vi "Main.vi"() -> ()   [LabVIEW 2015]
doc: "本模板用于队列消息处理器设计模式。\n\n事件处理循环负责按用户界面操作生成对应的消息。\n\n消息处理循环负责对事件处理循环或其他消息生成的消息进行处理。消息内容为字符串值，因此很容易将新消息添加至“消息处理”循环的“消息分支”条件结构。每个消息簇还可选择性地为消息数据提供一个变体，变体数据可以转换为消息数据所需要的任意类型。"
uses:
  controls/UI Data.ctl
  <vilib>/Platform/TimedLoop/XDataNode/timing_clust.ctl
  <vilib>/Platform/TimedLoop/XDataNode/nitl_modes.ctl
  <vilib>/Platform/TimedLoop/XDataNode/wakeup.ctl
  support/Message Queue/Enqueue Message (Single).vi
  <vilib>/Utility/file.llb/Read Delimited Spreadsheet (string).vi
  <vilib>/Utility/error.llb/Error Cluster From Error Code.vi
  <vilib>/Platform/TimedLoop/XDataNode/XDataNode.xnode
  <vilib>/ErrorRing/Error Ring.xnode
  support/Message Queue/Message Queue.lvlib
  support/User Event - Stop/User Event - Stop.lvlib
  <vilib>/Platform/TimedLoop/XDataNode/XDNodeRunTimeDep.lvlib
panel:
  in  "选项卡控件":enum32{"总线检查", "报告生成"}(tab)
  in  "总线检查":bool
  in  "1560":refnum<visa-resource-name>="COM3"
  in  "目标温度":string(combo)
  in  "样品编号":string
  in  "生成报告":bool
  in  "误差计算":bool
  in  "均匀性测量":bool
  in  "位置":enum16{"A", "B", "C", "D", "E", "F", "G", "H"}(ring)
  in  "均匀性表格":string[][](table)=[["A", "O", "E", "O"], ["", "", "", ""], ["", "", "", ""], ["", "", "", ""], ["", "", "", ""], ["", "", "", ""], ["", "", "", ""], ["B", "O", "F", "O"], ["", "", "", ""], ["", "", "", ""], ["", "", "", ""], ["", "", "", ""], ["", "", "", ""], ["", "", "", ""], ["C", "O", "G", "O"], ["", "", "", ""], ["", "", "", ""], ["", "", "", ""], ["", "", "", ""], ["", "", "", ""], ["", "", "", ""], ["D", "O", "H", "O"], ["", "", "", ""], ["", "", "", ""], ["", "", "", ""], ["", "", "", ""], ["", "", "", ""], ["", "", "", ""], ["", "", "", ""], ["", "", "", ""]]
  in  "波动性表格":string[][](table)
  out "显示<替换该项>":string
  in  "波动性测量":bool
  in  "退出":bool
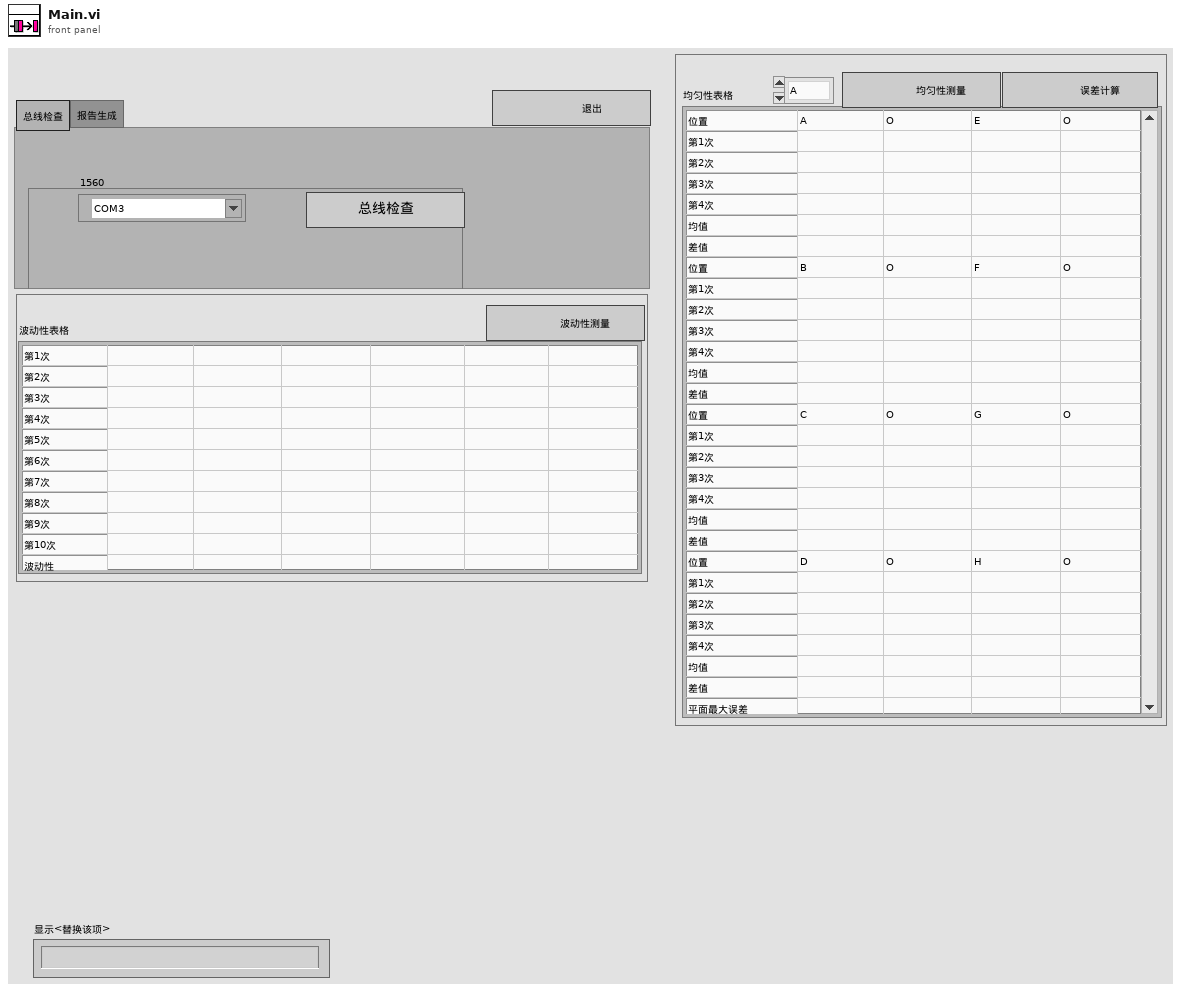
[diagram p1: front panel]
types:
  T1 = typedef "UI Data.ctl" = cluster{"布尔<替换该项>":bool, "字符串<替换该项>":string, "数值<替换该项>":dbl, "执行某操作引用":refnum<vi>, "执行其他操作引用":refnum<vi>, "数据显示引用":refnum<vi>, "退出按钮引用":refnum<vi>}
  T2 = typedef "Message Queue.lvlib/All Message Queues.ctl" = cluster{"UI":refnum<queue>}
  T3 = cluster{"Baud Rate (9600)":u32, "Flow Control (1: XON/XOFF)":u16, "Termination Char (0:CR)":u16}
  T4 = typedef "XDNodeRunTimeDep.lvlib/timing_clust.ctl" = cluster{"Expected End [f-1]":u64, "Actual End [f-1]":u64, "Finished Late? [f-1]":bool, "Expected End [i-1]":u64, "Actual End [i-1]":u64, "Finished Late? [i-1]":bool, "Expected Start [i]":u64, "Actual Start [i]":u64, "Expected Start [f]":u64, "Actual Start [f]":u64, "Source Name":string, "Structure Name":string, "Period":i64, "Deadline":i64, "Offset":i64, "Start":i64, "Priority":i32, "Timeout":i32, "Mode":T5, "Wakeup Reason":T6, "Error":errorcluster, "Source Type":string, "Secondary Source Type":string, "Global End Time":u64, "Global Start Time":u64, "Frame Duration":u64, "Iteration Duration":u64, "Assigned CPU":i32, "I/O Scan Engine Mode":u32}
  T5 = typedef "XDNodeRunTimeDep.lvlib/nitl_modes.ctl" = enum32{"No Change", "Process missed periods, maintain original phase", "Discard missed periods, maintain original phase", "Process missed periods, ignore original phase", "Discard missed periods, ignore original phase"}
  T6 = typedef "XDNodeRunTimeDep.lvlib/wakeup.ctl" = enum32{"Normal", "Aborted", "Asynchronous wakeup", "Timing source error", "Timed loop error", "Timeout"}
  T7 = enum8{"Enabled", "Disabled", "Disabled and Grayed Out"}
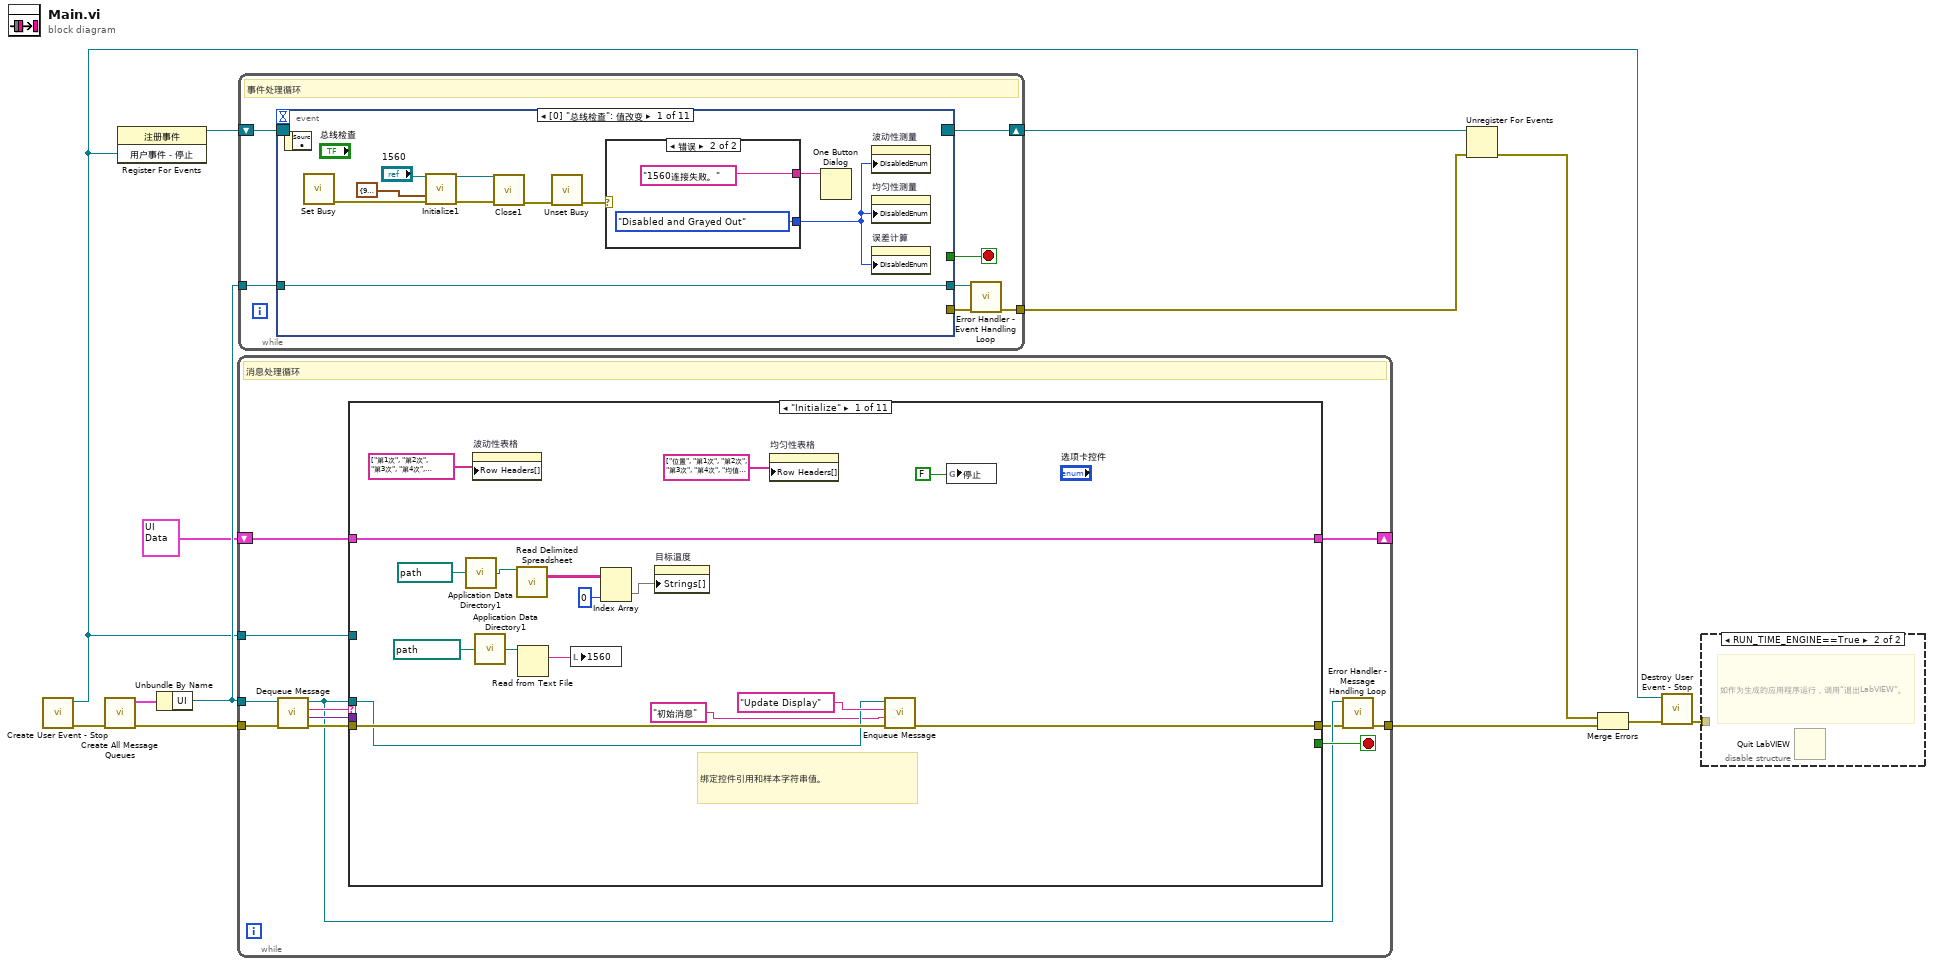
[diagram p0: block diagram]
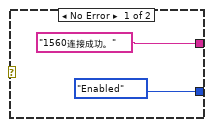
[diagram p3: hidden frame]
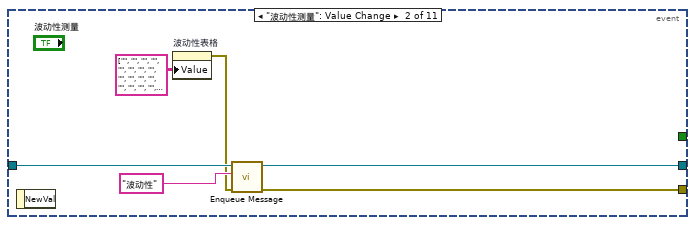
[diagram p4: hidden frame]
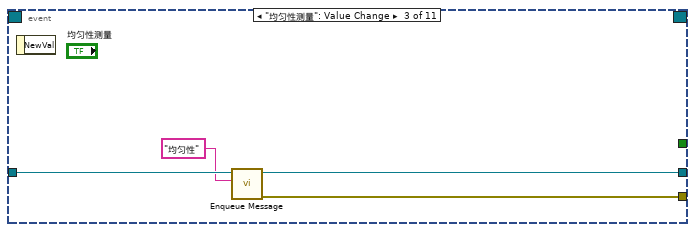
[diagram p5: hidden frame]
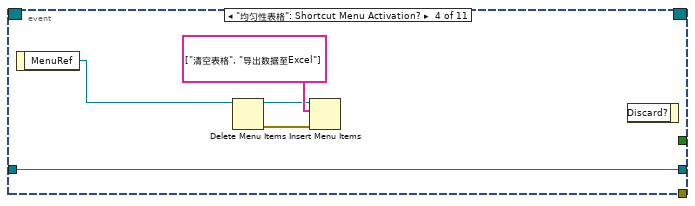
[diagram p6: hidden frame]
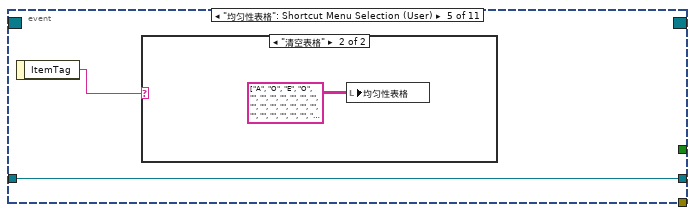
[diagram p7: hidden frame]
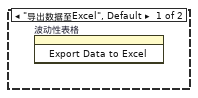
[diagram p8: hidden frame]
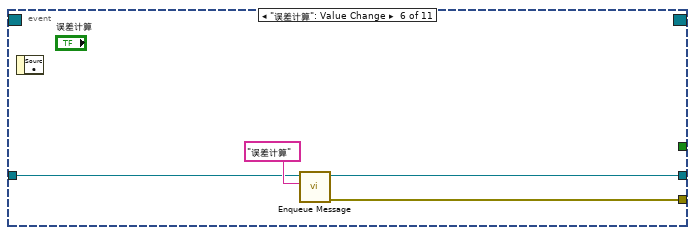
[diagram p9: hidden frame]
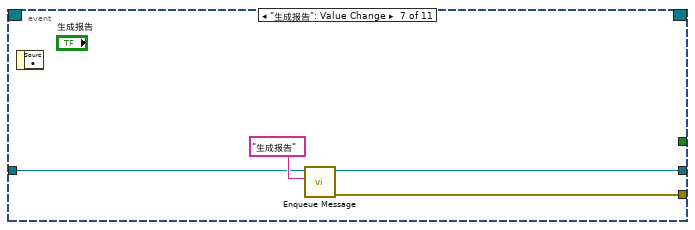
[diagram p10: hidden frame]
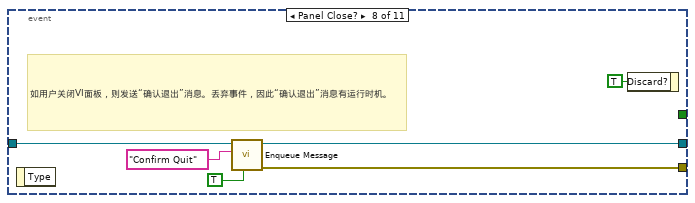
[diagram p11: hidden frame]
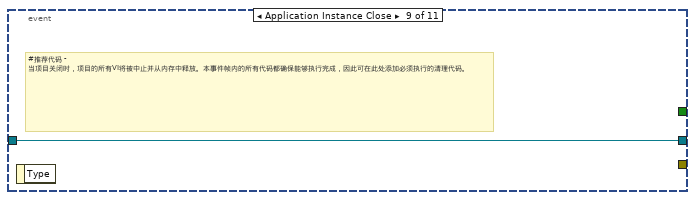
[diagram p12: hidden frame]
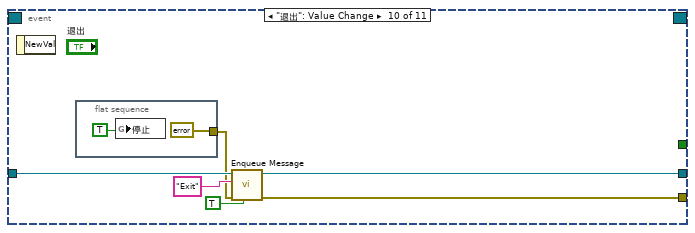
[diagram p13: hidden frame]
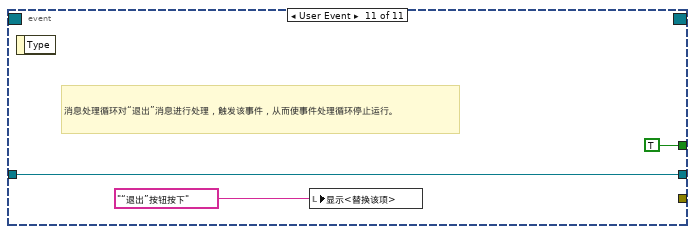
[diagram p14: hidden frame]
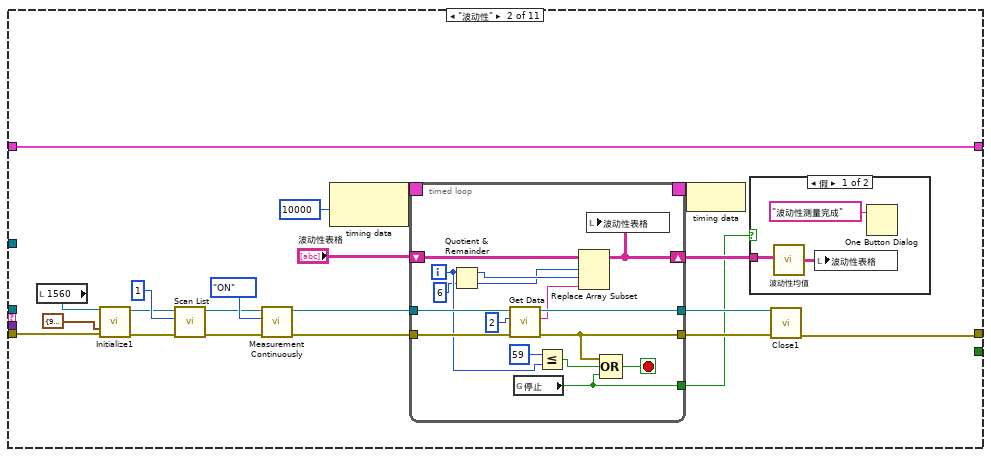
[diagram p15: hidden frame]
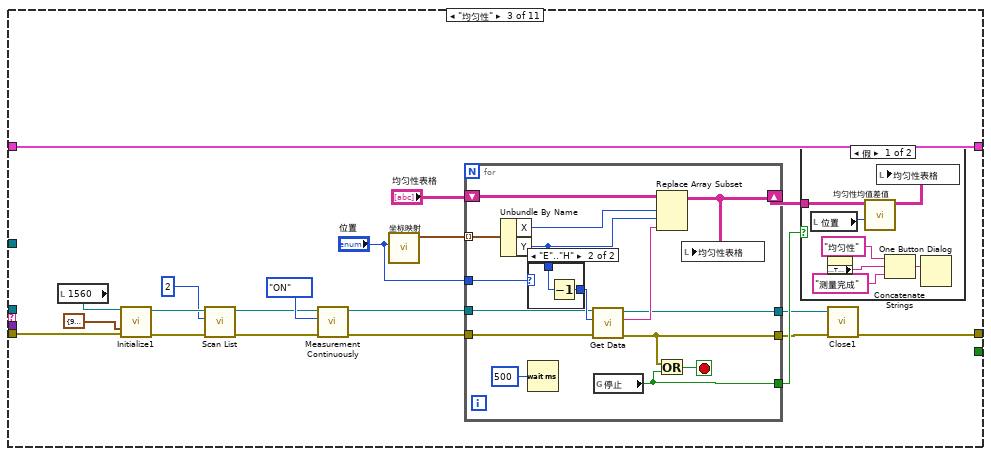
[diagram p17: hidden frame]
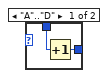
[diagram p19: hidden frame]
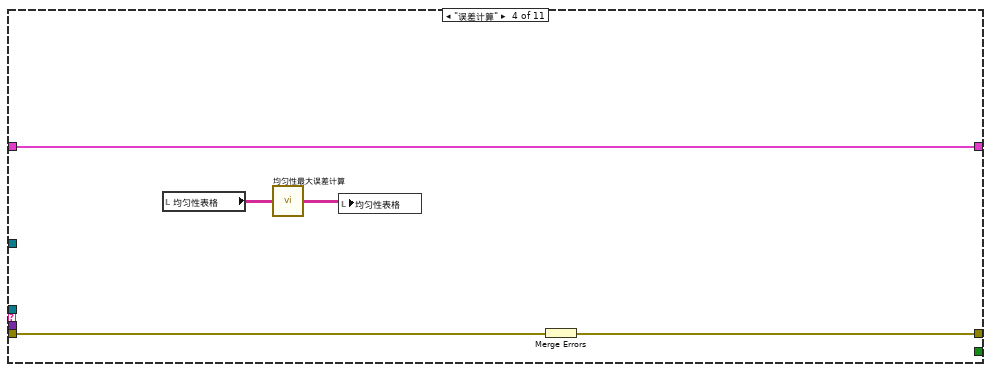
[diagram p20: hidden frame]
diagram:
  n1 = call "Create User Event - Stop.vi"() -> ("error out"=w9:cluster{"状态":bool, "代码":i32, "源":string}, "用户事件－停止"=w1:refnum<user-event>)  [unwired: 10 in]
  n2 = call "Create All Message Queues.vi"("error in (no error)"=w9) -> ("error out"=w13:cluster{"状态":bool, "代码":i32, "源":string}, "消息队列输出"=w12:T2)  [unwired: 9 in]
  n3 = register-events(w1) -> (reference out=w2:refnum<event-registration>)  [unwired: 2 in, 1 out]
  n4 = Unbundle By Name(w12) -> ("UI"=w10:refnum<queue>)
  n5 = while {
    tunnel: w10 -> [w17]
    shift-right: [w24] -> _
    shift-left: T1 {"布尔<替换该项>"=FALSE, "字符串<替换该项>"="", "数值<替换该项>"=0.0, "执行某操作引用"=refnum, "执行其他操作引用"=refnum, "数据显示引用"=refnum, "退出按钮引用"=refnum} ("Data Cluster") -> [w25]
    tunnel: w1 -> [w22]
    tunnel: w13 -> [w21]
    tunnel: [w15] -> w11
    stop <- w23 stop-if-true
    # "消息处理循环"
    n6 = call "Dequeue Message.vi"("error in (no error)"=w21, "消息队列"=w17) -> ("error out"=w20:cluster{"状态":bool, "代码":i32, "源":string}, "消息数据"=w18:variant, "消息"=w19:string, "消息队列副本"=w16:refnum<queue>)  [unwired: 6 in]
    n7 = case "消息分支" shown="\"Initialize\"" w19 {
      selector: w19 -> [_ _ _ _ _ _ _ _ _ _ w200]
      tunnel: w16 -> [w39 _ _ _ _ _ _ w181 _ w199 _]
      tunnel: w20 -> [w41 w48 w99 w139 w140 w169 w178 w185 w188 w192 _]
      tunnel: [w42 w47 w90 w137 w142 w170 w172 w183 w186 w195 w201] -> w14
      tunnel: w25 -> [w31 w63 w108 w138 w149 w171 w177 w184 w187 w198 w202]
      tunnel: [w31 w63 w108 w138 w149 w171 w177 w184 w187 w198 w202] -> w24
      tunnel: [_ _ _ _ _ _ _ _ _ TRUE _] -> w23
      tunnel: w18 -> [_ _ _ _ _ w168 w176 _ _ w189 _]
      tunnel: w22 -> [_ _ _ _ _ _ _ _ _ w194 _]
      frame "Initialize" {
        # "绑定控件引用和样本字符串值。"
        # "初始化 - 全部初始化工作应开始于此消息，因其他循环可能立即将在此消息后执行的消息加至队列。"
        n8 = call "Application Data Directory1.vi"("Relative path (.)"=path "温度.txt") -> ("Application Directory (+ Relative)"=w28:path)
        n9 = property on="波动性表格" class="Tbl (严格)"("Row Headers[]"=string[] ["第1次", "第2次", "第3次", "第4次", "第5次", "第6次", "第7次", "第8次", "第9次", "第10次", "波动性"] ("行首字符串[]")) -> ()  [unwired: 2 in, 2 out]
        n10 = call "Application Data Directory1.vi"("Relative path (.)"=path "串口号.txt") -> ("Application Directory (+ Relative)"=w26:path)
        n11 = call-poly <vilib>:"Read Delimited Spreadsheet.vi"("file path (dialog if empty)"=w28) -> ("all rows"=w33:string[][])  [unwired: 9 in, 5 out]
        n12 = Read from Text File(file (use dialog)=w26) -> (text=w30:string)  [unwired: 3 in, 3 out]
        n13 = local write "1560"(w30) -> ()
        n14 = Index Array(array=w33, index (col)=0 ("禁用的索引 (列)")) -> (element=w32:string[])  [unwired: 1 in]
        n15 = property on="目标温度" class="CmbBox"("Strings[]"=w32) -> ()  [unwired: 2 in, 2 out]
        n16 = property on="均匀性表格" class="Tbl (严格)"("Row Headers[]"=string[] ["位置", "第1次", "第2次", "第3次", "第4次", "均值", "差值", "位置", "第1次", "第2次", "第3次", "第4次", "均值", "差值", "位置", "第1次", "第2次", "第3次", "第4次", "均值", "差值", "位置", "第1次", "第2次", "第3次", "第4次", "均值", "差值", "平面最大误差", "工作区域最大误差"] ("行首字符串[]")) -> ()  [unwired: 2 in, 2 out]
        n17 = call-poly "Enqueue Message.vi"("error in (no error)"=w41, "消息数据"="初始消息" ("Initial Message"), "消息"="Update Display" ("Message"), "消息队列"=w39) -> ("error out"=w42:cluster{"状态":bool, "代码":i32, "源":string})  [unwired: 6 in, 1 out]
        n18 = global write "全局.vi" "停止"(FALSE ("停止")) -> ()
      }
      frame "波动性" {
        # "Something - 将该消息自行替换为应用程序需要的消息。"
        n19 = local read "1560"() -> (w55:refnum<visa-resource-name>)
        n20 = call "Initialize1.vi"("VISA resource name"=w55, "Serial Configuration"=T3 {"Baud Rate (9600)"=9600, "Flow Control (1: XON/XOFF)"=1, "Termination Char (0:CR)"=0}, "error in (no error)"=w48) -> ("VISA resource name out"=w58:refnum<visa-resource-name>, "error out"=w57:errorcluster)  [unwired: 11 in]
        n21 = call "Scan List.vi"("error in (no error)"=w57, "通道数"=1 ("通道号"), "VISA resource name"=w58) -> ("error out"=w59:errorcluster, "VISA resource name out"=w60:refnum<visa-resource-name>)  [unwired: 7 in]
        n22 = call "Measurement Continuously.vi"("error in (no error)"=w59, "开关"=enum16{"OFF", "ON"}."ON", "VISA resource name"=w60) -> ("error out"=w50:errorcluster, "VISA resource name out"=w49:refnum<visa-resource-name>)  [unwired: 7 in]
        n23 = node-c288(i64 10000 ("周期")) -> (w54:T4)
        n24 = timed-loop {
          timing: w54 -> [_]
          timing-out: [_] -> w53
          tunnel: w50 -> [w82]
          tunnel: w49 -> [w81]
          tunnel: [w80] -> w51
          tunnel: [w69] -> w52
          shift-right: [w71] -> w44
          shift-left: "波动性表格" -> [w77]
          tunnel: [w67] -> w43
          i -> [w75]
          stop <- w70 stop-if-true
          n25 = Quotient & Remainder(x=w75, y=6) -> (x-y*floor(x/y)=w73:i32, floor(x/y)=w72:i32)
          n26 = call "Get Data.vi"("error in (no error)"=w82, "通道号"=2, "VISA resource name"=w81) -> ("error out"=w69:errorcluster, "读取缓冲区"=w76:string, "VISA resource name out"=w80:refnum<visa-resource-name>)  [unwired: 6 in]
          n27 = global read "全局.vi" "停止"() -> (w67:bool)
          n28 = Less Or Equal?(x=59, y=w75) -> (x <= y?=w68:bool)
          n29 = Replace Array Subset(array=w77, new element=w76, index (row)=w72, index (col)=w73) -> (w71:string[][])
          n30 = local write "波动性表格"(w71) -> ()
          n31 = Compound Arithmetic op=OR ("复合运算")(w69, w68, w67) -> (w70:bool)
        }
        n32 = node-c288(w53) -> ()
        n33 = case shown="假" w43 {
          tunnel: w44 -> [w66 _]
          frame False {
            n34 = call "波动性均值.vi"("波动性表格"=w66) -> ("波动性表格1"=w65:string[][])
            n35 = local write "波动性表格"(w65) -> ()
            n36 = One Button Dialog(message="波动性测量完成" ("消息")) -> ()  [unwired: 1 in, 1 out]
          }
          frame True {
          }
        }
        n37 = call "Close1.vi"("VISA resource name"=w51, "error in (no error)"=w52) -> ("error out"=w47:errorcluster)  [unwired: 13 in]
      }
      frame "均匀性" {
        # "Something Else - 将该消息自行替换为应用程序需要的消息。"
        n38 = local read "1560"() -> (w100:refnum<visa-resource-name>)
        n39 = call "Initialize1.vi"("VISA resource name"=w100, "Serial Configuration"=T3 {"Baud Rate (9600)"=9600, "Flow Control (1: XON/XOFF)"=1, "Termination Char (0:CR)"=0}, "error in (no error)"=w99) -> ("VISA resource name out"=w103:refnum<visa-resource-name>, "error out"=w102:errorcluster)  [unwired: 11 in]
        n40 = call "Scan List.vi"("error in (no error)"=w102, "通道数"=2 ("通道号"), "VISA resource name"=w103) -> ("error out"=w104:errorcluster, "VISA resource name out"=w105:refnum<visa-resource-name>)  [unwired: 7 in]
        n41 = call "Measurement Continuously.vi"("error in (no error)"=w104, "开关"=enum16{"OFF", "ON"}."ON", "VISA resource name"=w105) -> ("error out"=w97:errorcluster, "VISA resource name out"=w98:refnum<visa-resource-name>)  [unwired: 7 in]
        n42 = call "坐标映射.vi"("位置"="位置") -> ("位置坐标"=w107:cluster{"X":i32, "Y":i32}[])  [unwired: 7 in, 3 out]
        n43 = for {
          tunnel: w107 -> [w126] mode=indexing
          tunnel: w98 -> [w128]
          tunnel: w97 -> [w129]
          shift-right: [w121] -> w96
          shift-left: "均匀性表格" -> [w127]
          tunnel: [w122] -> w91
          tunnel: [w119] -> w93
          tunnel: [w118] -> w92
          tunnel: "位置" -> [w117]
          stop <- w123 stop-if-true
          n44 = Unbundle By Name(w126) -> ("X"=w125:i32, "Y"=w120:i32)
          n45 = case shown="\"E\"..\"H\"" w117 {
            tunnel: [w132 w134] -> w130
            tunnel: w120 -> [w131 w133]
            frame "A".."D" {
              n46 = Increment(x=w131) -> (x+1=w132:i32)
            }
            frame "E".."H" {
              n47 = Decrement(x=w133) -> (x-1=w134:i32)
            }
          }
          n48 = Wait (ms)(milliseconds to wait=u32 500 ("等待时间（毫秒）")) -> ()  [unwired: 1 out]
          n49 = call "Get Data.vi"("error in (no error)"=w129, "通道号"=w130, "VISA resource name"=w128) -> ("error out"=w122:errorcluster, "读取缓冲区"=w124:string, "VISA resource name out"=w118:refnum<visa-resource-name>)  [unwired: 6 in]
          n50 = global read "全局.vi" "停止"() -> (w119:bool)
          n51 = Replace Array Subset(array=w127, new element=w124, index (row)=w125, index (col)=w120) -> (w121:string[][])
          n52 = Or(x=w122, y=w119) -> (x .or. y?=w123:bool)
          n53 = local write "均匀性表格"(w121) -> ()
        }
        n54 = case shown="假" w93 {
          tunnel: w96 -> [w115 _]
          frame False {
            n55 = local read "位置"() -> (w114:enum16{"A", "B", "C", "D", "E", "F", "G", "H"})
            n56 = property on="位置" class="Enum (严格)"() -> ("RingText.Text"=w111:string)  [unwired: 2 in, 2 out]
            n57 = call "均匀性均值差值.vi"("位置"=w114, "均匀性表格"=w115) -> ("输出数组"=w113:string[][])  [unwired: 9 in]
            n58 = local write "均匀性表格"(w113) -> ()
            n59 = Concatenate Strings("均匀性" ("消息"), w111, "测量完成" ("消息")) -> (w109:string)
            n60 = One Button Dialog(message=w109) -> ()  [unwired: 1 in, 1 out]
          }
          frame True {
          }
        }
        n61 = call "Close1.vi"("VISA resource name"=w92, "error in (no error)"=w91) -> ("error out"=w90:errorcluster)  [unwired: 13 in]
      }
      frame "误差计算" {
        # "如需创建新消息，可创建该帧的副本。在副本中，将本注释更改为对应消息的注释。"
        n62 = local read "均匀性表格"() -> (w136:string[][])
        n63 = call "均匀性最大误差计算.vi"("均匀性表格"=w136) -> ("输出数组"=w135:string[][])
        n64 = local write "均匀性表格"(w135) -> ()
        n65 = Merge Errors(w139) -> (w137:errorcluster)
      }
      frame "生成报告" {
        # "如需创建新消息，可创建该帧的副本。在副本中，将本注释更改为对应消息的注释。"
        n66 = Empty String/Path?(string/path="样品编号") -> (empty?=w146:bool)
        n67 = Empty String/Path?(string/path="目标温度") -> (empty?=w145:bool)
        n68 = call <vilib>:"Set Busy.vi"("error in (no error)"=w140) -> ("error out"=w141:errorcluster)  [unwired: 9 in, 1 out]
        n69 = Or(x=w146, y=w145) -> (x .or. y?=w144:bool)
        n70 = case shown="假" w144 {
          tunnel: "样品编号" -> [w153 _]
          tunnel: "目标温度" -> [w152 _]
          tunnel: w141 -> [w151 w163]
          tunnel: [w150 w163] -> w143
          frame False {
            n71 = call "原始记录路径.vi"("目标温度"=w152, "文件夹名称"=w153) -> ("file exists?"=w155:bool, "保存路径"=w154:path)  [unwired: 8 in]
            n72 = case shown="假" w155 {
              tunnel: w154 -> [w161 _]
              tunnel: w153 -> [w158 _]
              tunnel: w152 -> [w157 _]
              tunnel: w151 -> [w156 w162]
              tunnel: [w156 w162] -> w150
              frame False {
                n73 = local read "波动性表格"() -> (w159:string[][])
                n74 = local read "均匀性表格"() -> (w160:string[][])
                n75 = call "生成报告.vi"("目标温度"=w157, "样品编号"=w158, "均匀性表格"=w160, "波动性表格"=w159, "原始记录路径"=w161) -> ()  [unwired: 7 in]
              }
              frame True {
              }
            }
          }
          frame True {
            n76 = One Button Dialog(message="样品编号与目标编号不能为空。" ("消息")) -> ()  [unwired: 1 in, 1 out]
          }
        }
        n77 = call <vilib>:"Unset Busy.vi"("error in (no error)"=w143) -> ("error out"=w142:errorcluster)  [unwired: 10 in]
      }
      frame "Update Display" {
        # "#推荐代码 - 如希望降低“消息处理循环”和用户界面之间的耦合度，可创建用户事件（类似本VI中的“停止”事件）－当用户界面需要更新时，通过用户事件向“事件处理循环”发送消息。"
        # "更新显示－将消息数据转换为字符串，显示在“数据显示”显示控件中。"
        n78 = Variant To Data(error in=w169, type="", Variant=w168) -> (data=→"显示<替换该项>":string, error out=w166:errorcluster)
        n79 = Merge Errors(w166) -> (w170:errorcluster)
      }
      frame "Error" {
        # "#推荐代码 - 如更改“错误”消息的名称，则必须同时在Check Loop Error.vi中更新消息的名称。"
        # "#推荐代码 - 考虑创建用于记录错误的系统。此错误仅做通知目的。须在产生错误的消息帧内处理特定错误。"
        # "错误 - 显示错误对话框。本应用程序中，该消息由每个循环结束处的“错误处理”VI发送。"
        n80 = Variant To Data(error in=w178, type=errorcluster {"status"=FALSE, "code"=0, "source"=""} ("error constant"), Variant=w176) -> (data=w174:errorcluster, error out=w173:errorcluster)
        n81 = call <vilib>:"Simple Error Handler.vi"("error in (no error)"=w174) -> ()  [unwired: 4 in, 5 out]
        n82 = Merge Errors(w173) -> (w172:errorcluster)
      }
      frame "Confirm Quit" {
        # "#添加代码 - 应用程序退出前，如需弹出“是否确定”提示框（或其他提示），请在此处添加代码。该消息通常由“面板关闭？”事件发送。"
        # "Confirm Quit - 该消息用于确认用户是否需要退出应用程序。"
        n83 = call-poly "Enqueue Message.vi"("优先消息？ (F)"=TRUE ("Priority Message? (F)"), "error in (no error)"=w185, "消息"="Exit" ("Message"), "消息队列"=w181) -> ("error out"=w182:cluster{"状态":bool, "代码":i32, "源":string})  [unwired: 6 in, 1 out]
        n84 = Merge Errors(w182) -> (w183:errorcluster)
      }
      frame "---Copy This Frame---" {
        # "如需创建新消息，可创建该帧的副本。在副本中，将本注释更改为对应消息的注释。"
        n85 = Merge Errors(w188) -> (w186:errorcluster)
      }
      frame "Exit" {
        # "停止VI"
        # "释放消息队列引用"
        # "#添加代码 - 此处按需要添加清理代码。注意，如果'退出' 作为错误结果被调用，则将显示错误对话框。为“退出”条件添加自定义错误处理。"
        # "退出 - 退出应用程序。"
        n86 = Variant To Data(type=errorcluster {"status"=FALSE, "code"=0, "source"=""} ("error constant"), Variant=w189) -> (data=w190:errorcluster)  [unwired: 1 in, 1 out]
        n87 = call <vilib>:"Simple Error Handler.vi"("error in (no error)"=w190) -> ()  [unwired: 4 in, 5 out]
        n88 = call "Fire User Event - Stop.vi"("用户事件－停止"=w194) -> ("error out"=w193:cluster{"状态":bool, "代码":i32, "源":string})  [unwired: 10 in]
        n89 = Release Queue(queue=w199, error in (no error)=w192) -> (error out=w196:errorcluster)  [unwired: 1 in, 2 out]
        n90 = Merge Errors(w193, w196) -> (w195:errorcluster)
      }
      frame Default {
        # "如得到的消息未经任何分支定义，则运行“默认”分支。输出程序错误。"
        n91 = xnode ("Error Ring")("参数 0"=w200) -> ("错误输出"=w201:errorcluster)
      }
    }
    n92 = call "Error Handler - Message Handling Loop.vi"("error in (no error)"=w14, "消息队列"=w16) -> ("错误输入副本"=w15:cluster{"状态":bool, "代码":i32, "源":string})  [unwired: 8 in, 1 out]
  }
  n93 = while {
    tunnel: w10 -> [w216]
    shift-right: [w214] -> w6
    shift-left: w2 -> [w215]
    tunnel: [w210] -> w3
    stop <- w212 stop-if-true
    # "事件处理循环"
    n94 = event shown="[0] \"总线检查\": 值改变" {
      selector: w215 -> [_ _ _ _ _ _ _ _ _ _ _]
      dyn-events: [_ _ _ _ _ _ _ _ _ _ _] -> w214
      timeout: _ -> [_ _ _ _ _ _ _ _ _ _ _]
      tunnel: [_ _ _ _ _ _ _ _ _ _ TRUE ("Discard?")] -> w212
      tunnel: w216 -> [w226 w236 w240 w245 w247 w251 w255 w261 w263 w269 w274]
      tunnel: [_ w233 w237 _ _ w249 w253 w260 _ w268 _] -> w213
      tunnel: [w226 w235 w239 w245 w247 w250 w254 w259 w263 w267 w274] -> w211
      event "总线检查": Value Change {
        n95 = event-data() -> ()  [unwired: 1 in, 1 out]
        n96 = call <vilib>:"Set Busy.vi"() -> ("error out"=w220:errorcluster)  [unwired: 10 in, 1 out]
        n97 = call "Initialize1.vi"("VISA resource name"="1560", "Serial Configuration"=T3 {"Baud Rate (9600)"=9600, "Flow Control (1: XON/XOFF)"=1, "Termination Char (0:CR)"=0}, "error in (no error)"=w220) -> ("VISA resource name out"=w222:refnum<visa-resource-name>, "error out"=w221:errorcluster)  [unwired: 11 in]
        n98 = call "Close1.vi"("VISA resource name"=w222, "error in (no error)"=w221) -> ("error out"=w225:errorcluster)  [unwired: 13 in]
        n99 = call <vilib>:"Unset Busy.vi"("error in (no error)"=w225) -> ("error out"=w224:errorcluster)  [unwired: 10 in]
        n100 = case shown="错误" w224 {
          tunnel: ["1560连接成功。" ("消息") "1560连接失败。" ("消息")] -> w223
          tunnel: [T7."Enabled" ("禁用") T7."Disabled and Grayed Out" ("禁用")] -> w217
          frame No Error {
          }
          frame Error {
          }
        }
        n101 = One Button Dialog(message=w223) -> ()  [unwired: 1 in, 1 out]
        n102 = property on="波动性测量" class="Bool"("DisabledEnum"=w217) -> ()  [unwired: 2 in, 2 out]
        n103 = property on="均匀性测量" class="Bool"("DisabledEnum"=w217) -> ()  [unwired: 2 in, 2 out]
        n104 = property on="误差计算" class="Bool"("DisabledEnum"=w217) -> ()  [unwired: 2 in, 2 out]
      }
      event "波动性测量": Value Change {
        n105 = event-data() -> ()  [unwired: 1 in, 1 out]
        n106 = property on="波动性表格" class="Tbl (严格)"("Value"=string[][] [["", "", "", "", "", ""], ["", "", "", "", "", ""], ["", "", "", "", "", ""], ["", "", "", "", "", ""], ["", "", "", "", "", ""], ["", "", "", "", "", ""], ["", "", "", "", "", ""], ["", "", "", "", "", ""], ["", "", "", "", "", ""], ["", "", "", "", "", ""], ["", "", "", "", "", " "]] ("波动性表格")) -> (error out=w231:errorcluster)  [unwired: 2 in, 1 out]
        n107 = call-poly "Enqueue Message.vi"("error in (no error)"=w231, "消息"="波动性" ("Message"), "消息队列"=w236) -> ("error out"=w233:cluster{"状态":bool, "代码":i32, "源":string}, "消息队列副本"=w235:refnum<queue>)  [unwired: 7 in]
      }
      event "均匀性测量": Value Change {
        n108 = event-data() -> ()  [unwired: 1 in, 1 out]
        n109 = call-poly "Enqueue Message.vi"("消息"="均匀性" ("Message"), "消息队列"=w240) -> ("error out"=w237:cluster{"状态":bool, "代码":i32, "源":string}, "消息队列副本"=w239:refnum<queue>)  [unwired: 8 in]
      }
      event "均匀性表格": Shortcut Menu Activation? {
        n110 = event-data() -> ("MenuRef"=w241:refnum<k9>)  [unwired: 1 in]
        n111 = Delete Menu Items(9:w241) -> (0:w242:errorcluster, 3:w243:refnum<k9>)  [unwired: 3 in]
        n112 = Insert Menu Items(6:w242, 8:string[] ["清空表格", "导出数据至Excel"] ("项名称"), 9:w243) -> ()  [unwired: 3 in, 3 out]
        n113 = event-data() -> ()  [unwired: 2 in, 1 out]
      }
      event "均匀性表格": Shortcut Menu Selection (User) {
        n114 = event-data() -> ("ItemTag"=w246:string)  [unwired: 1 in]
        n115 = case shown="\"清空表格\"" w246 {
          frame "导出数据至Excel", Default {
            n116 = invoke on="波动性表格" class="Tbl (严格)" method="Export Data to Excel"() -> ()  [unwired: 3 in, 3 out]
          }
          frame "清空表格" {
            n117 = local write "均匀性表格"(string[][] [["A", "O", "E", "O"], ["", "", "", ""], ["", "", "", ""], ["", "", "", ""], ["", "", "", ""], ["", "", "", ""], ["", "", "", ""], ["B", "O", "F", "O"], ["", "", "", ""], ["", "", "", ""], ["", "", "", ""], ["", "", "", ""], ["", "", "", ""], ["", "", "", ""], ["C", "O", "G", "O"], ["", "", "", ""], ["", "", "", ""], ["", "", "", ""], ["", "", "", ""], ["", "", "", ""], ["", "", "", ""], ["D", "O", "H", "O"], ["", "", "", ""], ["", "", "", ""], ["", "", "", ""], ["", "", "", ""], ["", "", "", ""], ["", "", "", ""], ["", "", "", ""], ["", "", "", ""]] ("均匀性表格")) -> ()
          }
        }
      }
      event "误差计算": Value Change {
        n118 = event-data() -> ()  [unwired: 1 in, 1 out]
        n119 = call-poly "Enqueue Message.vi"("消息"="误差计算" ("Message"), "消息队列"=w251) -> ("error out"=w249:cluster{"状态":bool, "代码":i32, "源":string}, "消息队列副本"=w250:refnum<queue>)  [unwired: 8 in]
      }
      event "生成报告": Value Change {
        n120 = event-data() -> ()  [unwired: 1 in, 1 out]
        n121 = call-poly "Enqueue Message.vi"("消息"="生成报告" ("Message"), "消息队列"=w255) -> ("error out"=w253:cluster{"状态":bool, "代码":i32, "源":string}, "消息队列副本"=w254:refnum<queue>)  [unwired: 8 in]
      }
      event Panel Close? {
        # "如用户关闭VI面板，则发送“确认退出”消息。丢弃事件，因此“确认退出”消息有运行时机。"
        n122 = event-data() -> ()  [unwired: 1 in, 1 out]
        n123 = call-poly "Enqueue Message.vi"("优先消息？ (F)"=TRUE ("Priority Message? (F)"), "消息"="Confirm Quit" ("Message"), "消息队列"=w261) -> ("error out"=w260:cluster{"状态":bool, "代码":i32, "源":string}, "消息队列副本"=w259:refnum<queue>)  [unwired: 7 in]
        n124 = event-data ("Event Filter Node")("Discard?"=TRUE) -> ()  [unwired: 1 in, 1 out]
      }
      event Application Instance Close {
        # "#推荐代码 - 当项目关闭时，项目的所有VI将被中止并从内存中释放。本事件帧内的所有代码都确保能够执行完成，因此可在此处添加必须执行的清理代码。"
        n125 = event-data() -> ()  [unwired: 1 in, 1 out]
      }
      event "退出": Value Change {
        n126 = event-data() -> ()  [unwired: 1 in, 1 out]
        n127 = flat-sequence {
          tunnel: [errorcluster {"status"=FALSE, "code"=0, "source"=""} ("错误常量")] -> w264
          frame #0 {
            n128 = global write "全局.vi" "停止"(TRUE ("停止")) -> ()
          }
        }
        n129 = call-poly "Enqueue Message.vi"("优先消息？ (F)"=TRUE ("Priority Message? (F)"), "error in (no error)"=w264, "消息"="Exit" ("Message"), "消息队列"=w269) -> ("error out"=w268:cluster{"状态":bool, "代码":i32, "源":string}, "消息队列副本"=w267:refnum<queue>)  [unwired: 6 in]
      }
      event User Event {
        # "消息处理循环对“退出”消息进行处理，触发该事件，从而使事件处理循环停止运行。"
        n130 = event-data() -> ()  [unwired: 1 in, 1 out]
        n131 = local write "显示<替换该项>"("“退出”按钮按下" ("VI Stopped")) -> ()
      }
    }
    n132 = call "Error Handler - Event Handling Loop.vi"("error in (no error)"=w213, "消息队列"=w211) -> ("错误输入副本"=w210:cluster{"状态":bool, "代码":i32, "源":string})  [unwired: 8 in, 1 out]
  }
  n133 = Unregister For Events(event registration refnum=w6, error in=w3) -> (error out=w7:errorcluster)
  n134 = Merge Errors(w7, w11) -> (w8:errorcluster)
  n135 = call "Destroy User Event - Stop.vi"("error in (no error)"=w8, "用户事件－停止"=w1) -> ("error out"=w4:cluster{"状态":bool, "代码":i32, "源":string})  [unwired: 9 in]
  n136 = disable-structure "Conditional Disable Structure" shown="RUN_TIME_ENGINE==True" {
    disable-tunnel: w4 -> [_ _]
    frame condition #0 (active) {
    }
    frame condition #1 {
      # "如作为生成的应用程序运行，调用“退出LabVIEW”。"
      n137 = Quit LabVIEW() -> ()  [unwired: 1 in]
    }
  }
